vi "PCO_GetApertureF.vi"(8 "error in (no error)":errorcluster {"code" format="%x"}, 11 "hLens":u64) -> (0 "error out":errorcluster {"code" format="%x"}, 1 "dwfAperturePos":u32, 2 "ErrorMessage":i32 format="%x", 3 "hLens out":u64, 4 "dwflags":u32, 5 "wAperturePos":u16)   [LabVIEW 2020, in "SDK.lvlib" / "LensControl.lvlib"]
doc: "<b>Description:</b>\nGets the current aperture position of the lens control device in f/position * 10 (member of dwApertures)\nThe value returned is one of the members of the current dwApertures array.\nThe dwApertures array is reinitialized in case the zoom changes and either PCO_GetApertureF or PCO_SetApertureF are called.\nChanges in zoom will be shown in dwflagsout as LENSCONTROL_OUT_ZOOMHASCHANGED.\n\n<b>Supported camera type:</b>\npco.edge CLHS, pco.dimax cs\n\n<b>Descriptor dependency:</b>\nNone"
uses:
  LensControl.lvlib
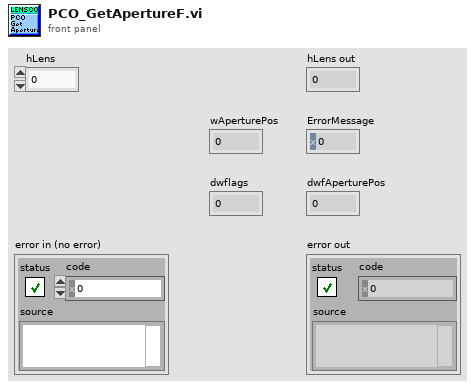
[diagram p1: front panel]
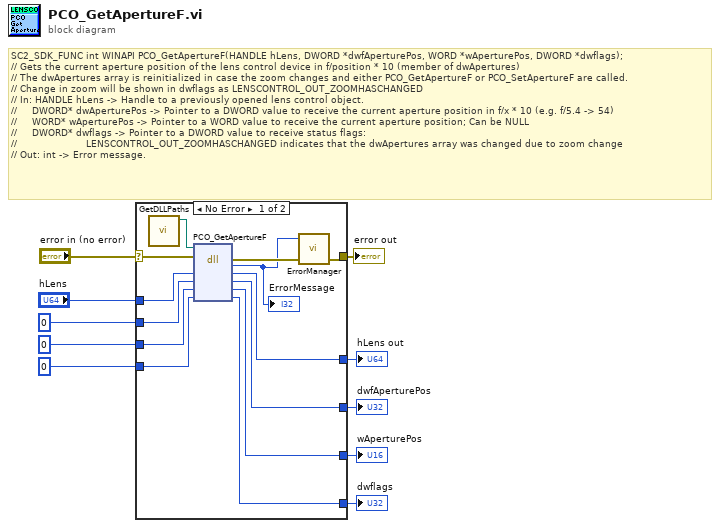
[diagram p0: block diagram]
diagram:
  # "SC2_SDK_FUNC int WINAPI PCO_GetApertureF(HANDLE hLens, DWORD *dwfAperturePos, WORD *wAperturePos, DWORD *dwflags);\n// Gets the current aperture position of the lens control device in f/position * 10 (member of dwApertures)\n// The dwApertures array is reinitialized in case the zoom changes and either PCO_GetApertureF or PCO_SetApertureF are called.\n// Change in zoom will be shown in dwflags as LENSCONTROL_OUT_ZOOMHASCHANGED\n// In: HANDLE hLens -> Handle to a previously opened lens control object.\n//     DWORD* dwAperturePos -> Pointer to a DWORD value to receive the current aperture position in f/x * 10 (e.g. f/5.4 -> 54)\n//     WORD* wAperturePos -> Pointer to a WORD value to receive the current aperture position; Can be NULL\n//     DWORD* dwflags -> Pointer to a DWORD value to receive status flags:\n//                       LENSCONTROL_OUT_ZOOMHASCHANGED indicates that the dwApertures array was changed due to zoom change\n// Out: int -> Error message."
  n1 = case shown="No Error" "error in (no error)" {
    selector: "error in (no error)" -> [w15 w28]
    tunnel: "hLens" -> [w23 w27]
    tunnel: [w22 w27] -> w9
    tunnel: u32 0 ("dwfAperturePos") -> [w21 w26]
    tunnel: [w20 w26] -> w7
    tunnel: u16 0 ("wAperturePos") -> [w19 w25]
    tunnel: [w18 w25] -> w5
    tunnel: u32 0 ("dwflags") -> [w17 w24]
    tunnel: [w16 w24] -> w3
    tunnel: [w14 w28] -> w2
    frame No Error {
      n2 = call "GetDLLPaths.vi"() -> ("SC2_Cam_Path"=w11:path)  [unwired: 9 in, 2 out]
      n3 = dll-call lib="?" fn="PCO_GetApertureF"(path in=w11, error in=w15, "hLens"=w23, "dwfAperturePos"=w21, "wAperturePos"=w19, "dwflags"=w17) -> (error out=w13:errorcluster, "return type"=w12:i32, "hLens"=w22:u64, "dwfAperturePos"=w20:u32, "wAperturePos"=w18:u16, "dwflags"=w16:u32)  [unwired: 1 in, 1 out]
      "ErrorMessage" <- w12
      n4 = call "ErrorManager.vi"("error in (no error)"=w13, "error code"=w12) -> ("error out"=w14:errorcluster)  [unwired: 3 in]
    }
    frame Error {
    }
  }
  "hLens out" <- w9
  "dwfAperturePos" <- w7
  "wAperturePos" <- w5
  "dwflags" <- w3
  "error out" <- w2
